vi "Initialize.vi"(8 "error in (no error)":errorcluster, 9 "Reset (True)":bool=TRUE, 10 "ID Query (True)":bool=TRUE, 11 "VISA resource name":refnum<visa-resource-name>) -> (0 "error out":errorcluster, 3 "VISA resource name out":refnum<visa-resource-name>)   [LabVIEW 2014, in "Agilent PSG MXG Series.lvlib"]
doc: "Establishes communication with the instrument and optionally performs an instrument identification query and/or an instrument reset. It also places the instrument in a default state needed for other instrument driver operations. Therefore, call this VI before calling other instrument driver VIs for this instrument. Generally, you need to call the <B>Initialize VI</B> only once at the beginning of an application."
uses:
  Agilent PSG MXG Series.lvlib
  Extended User Data.ctl
  Match Regular Expression.xnode
panel:
  # "(c) 2007-2015 National Instruments.  ALL RIGHTS RESERVED."
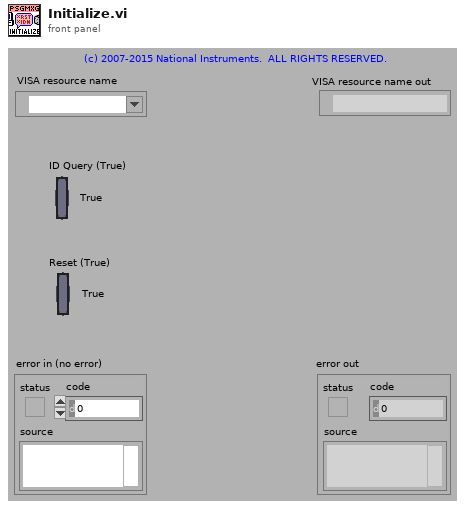
[diagram p1: front panel]
types:
  T1 = typedef "Agilent PSG MXG Series.lvlib/Extended User Data.ctl" = cluster{"Options":string[]}
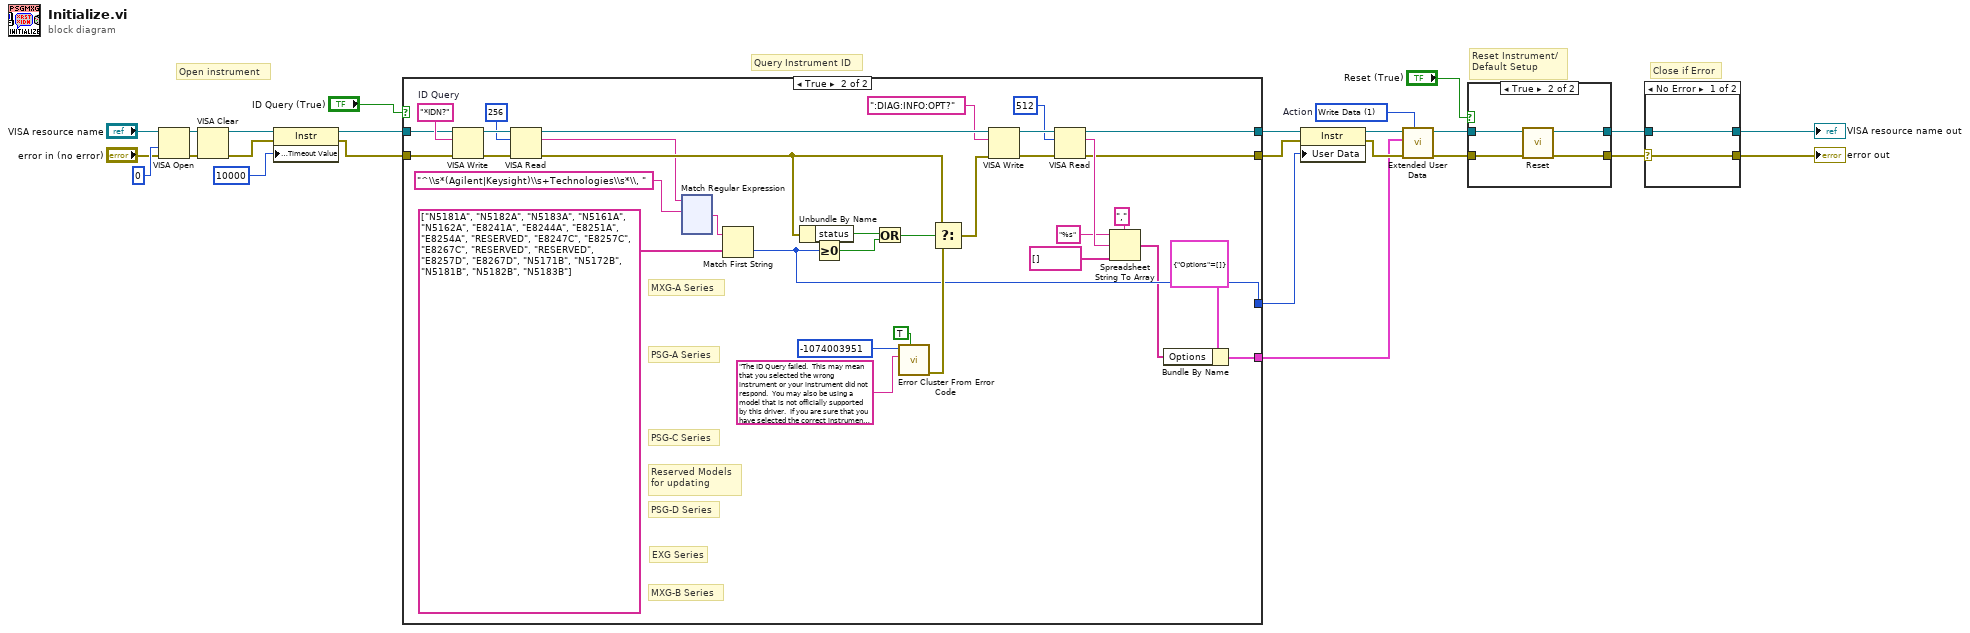
[diagram p0: block diagram]
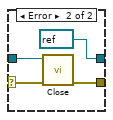
[diagram p2: hidden frame]
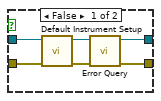
[diagram p3: hidden frame]
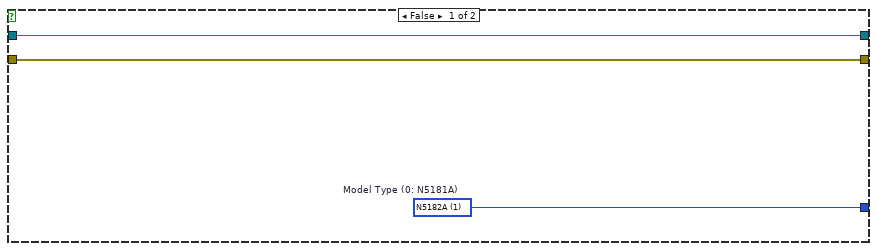
[diagram p4: hidden frame]
diagram:
  w4 = u16 1 items=["Read Data", "Write Data", "Clear Data", "Clear ALL Data"]  # Action
  # "Close if Error"
  # "Query Instrument ID"
  # "Reset Instrument/\nDefault Setup"
  # "Open instrument"
  n1 = VISA Open(access mode=u32 0, error in (no error)="error in (no error)", VISA resource name="VISA resource name") -> (VISA resource name=w23:refnum<visa-resource-name>, error out=w22:errorcluster)  [unwired: 2 out]
  n2 = VISA Clear(VISA resource name=w23, error in (no error)=w22) -> (VISA resource name out=w21:refnum<visa-resource-name>, error out=w20:errorcluster)
  n3 = property class="Instr"(reference=w21, error in=w20, "General Settings:Timeout Value"=u32 10000) -> (reference out=w8:refnum<visa-resource-name>, error out=w7:errorcluster)
  n4 = case shown="True" "ID Query (True)" {
    tunnel: [w27 w35] -> w16
    tunnel: [w28 w36] -> w17
    tunnel: [w26 w50] -> w15
    tunnel: w8 -> [w28 w48]
    tunnel: w7 -> [w27 w47]
    tunnel: [_ w32] -> w3
    frame False {
      w26 = u16 1 items=["N5181A"=0, "N5182A"=1, "N5183A"=2, "N5161A"=3, "N5162A"=4, "E8241A"=5, "E8244A"=6, "E8251A"=7, "E8254A"=8, "E8247C"=10, "E8257C"=11, "E8267C"=12, "E8257D"=15, "E8267D"=16, "N5171B"=17, "N5172B"=18, "N5181B"=19, "N5182B"=20]  # Model Type (0: N5181A)
    }
    frame True {
      w59 = "*IDN?"  # ID Query
      # "EXG Series"
      # "MXG-B Series"
      # "Reserved Models\nfor updating"
      # "PSG-D Series"
      # "PSG-C Series"
      # "PSG-A Series"
      # "MXG-A Series"
      n5 = VISA Write(VISA resource name=w48, write buffer=w59, error in (no error)=w47) -> (VISA resource name out=w62:refnum<visa-resource-name>, error out=w61:errorcluster)  [unwired: 1 out]
      n6 = VISA Read(VISA resource name=w62, byte count=u32 256, error in (no error)=w61) -> (VISA resource name out=w46:refnum<visa-resource-name>, read buffer=w30:string, error out=w54:errorcluster)  [unwired: 1 out]
      n7 = xnode ("Match Regular Expression")("input string"=w30, "regular expression"="^\\s*(Agilent|Keysight)\\s+Technologies\\s*\\, " ("Company Name Regular Expression")) -> ("after match"=w29:string)  [unwired: 4 in, 4 out]
      n8 = Match First String(2:string[] ["N5181A", "N5182A", "N5183A", "N5161A", "N5162A", "E8241A", "E8244A", "E8251A", "E8254A", "RESERVED", "E8247C", "E8257C", "E8267C", "RESERVED", "RESERVED", "E8257D", "E8267D", "N5171B", "N5172B", "N5181B", "N5182B", "N5183B"], 3:w29) -> (0:w50:i32)  [unwired: 1 out]
      n9 = Unbundle By Name(w54) -> ("status"=w53:bool)
      n10 = Greater Or Equal To 0?(x=w50) -> (x >= 0?=w51:bool)
      n11 = Or(x=w53, y=w51) -> (x .or. y?=w52:bool)
      n12 = call "Error Cluster From Error Code.vi"("show call chain? (False)"=TRUE, "error message (\"\")"="The ID Query failed.  This may mean that you selected the wrong instrument or your instrument did not respond.  You may also be using a model that is not officially supported by this driver.  If you are sure that you have selected the correct instrument and it is responding, try disabling the ID Query." ("Source (VI Name)"), "error code (0)"=-1074003951 ("Code")) -> ("error out"=w58:errorcluster)  [unwired: 1 in, 5 out]
      n13 = Select(t=w54, s=w52, f=w58) -> (s? t:f=w45:errorcluster)
      n14 = VISA Write(VISA resource name=w46, write buffer=":DIAG:INFO:OPT?", error in (no error)=w45) -> (VISA resource name out=w43:refnum<visa-resource-name>, error out=w42:errorcluster)  [unwired: 1 out]
      n15 = VISA Read(VISA resource name=w43, byte count=u32 512, error in (no error)=w42) -> (VISA resource name out=w36:refnum<visa-resource-name>, read buffer=w40:string, error out=w35:errorcluster)  [unwired: 1 out]
      n16 = Spreadsheet String To Array(delimiter (Tab)=",", format string="%s", spreadsheet string=w40, array type (2D Dbl)=string[] []) -> (array=w33:string[])
      n17 = Bundle By Name(cluster=T1 {"Options"=[]} ("User Data Out"), "Options"=w33) -> (w32:T1)
    }
  }
  n18 = property class="Instr"(reference=w17, error in=w16, "User Data"=w15) -> (reference out=w6:refnum<visa-resource-name>, error out=w5:errorcluster)
  n19 = call "Extended User Data.vi"("Action"=w4, "error in (no error)"=w5, "User Data In"=w3, "VISA resource name"=w6) -> ("error out"=w1:errorcluster, "VISA resource name out"=w2:refnum<visa-resource-name>)  [unwired: 6 out]
  n20 = case shown="True" "Reset (True)" {
    tunnel: w1 -> [w178 w180]
    tunnel: [w174 w183] -> w18
    tunnel: w2 -> [w179 w181]
    tunnel: [w175 w182] -> w19
    frame False {
      n21 = call "Default Instrument Setup.vi"("error in (no error)"=w178, "VISA resource name"=w179) -> ("error out"=w176:errorcluster, "VISA resource name out"=w177:refnum<visa-resource-name>)  [unwired: 8 out]
      n22 = call "Error Query.vi"("error in (no error)"=w176, "VISA resource name"=w177) -> ("error out"=w174:errorcluster, "VISA resource name out"=w175:refnum<visa-resource-name>)  [unwired: 8 out]
    }
    frame True {
      n23 = call "Reset.vi"("error in (no error)"=w180, "VISA resource name"=w181) -> ("error out"=w183:errorcluster, "VISA resource name out"=w182:refnum<visa-resource-name>)  [unwired: 8 out]
    }
  }
  n24 = case shown="No Error" w18 {
    selector: w18 -> [w184 w187]
    tunnel: w19 -> [w185 w188]
    tunnel: [w185 refnum<visa-resource-name> refnum ("VISA resource name out")] -> w10
    tunnel: [w184 w189] -> w9
    frame No Error {
    }
    frame Error {
      n25 = call "Close.vi"("error in (no error)"=w187, "VISA resource name"=w188) -> ("error out"=w189:errorcluster)  [unwired: 9 out]
    }
  }
  "VISA resource name out" <- w10
  "error out" <- w9
